vi "GT Axis Off.vi"(8 "error in (no error)":errorcluster caption="错误输入（无错误）", 10 "axis":i16, 11 "cardNum":i16) -> (0 "error out":errorcluster caption="错误输出", 3 "function return":i16)   [LabVIEW 2014, in "gts.lvlib"]
doc: "GT_API GT_AxisOff(short cardNum,short axis);"
uses:
  gts.lvlib
  gts.dll
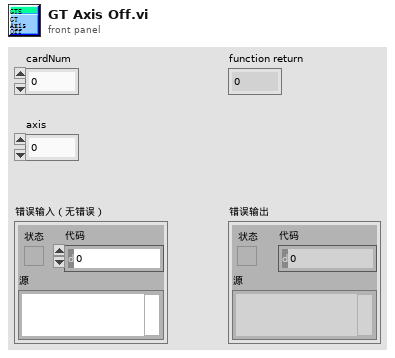
[diagram p1: front panel]
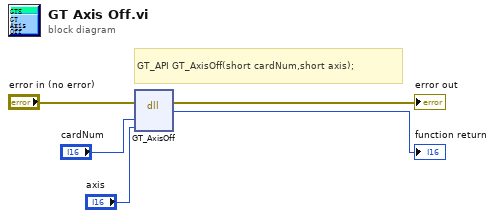
[diagram p0: block diagram]
diagram:
  # "GT_API GT_AxisOff(short cardNum,short axis);"
  n1 = dll-call lib="PTH2>abs F.多卡库-控制卡基本运动例程(labview)gts.*" fn="GT_AxisOff"(error in="error in (no error)", "cardNum"="cardNum", "axis"="axis") -> (error out=→"error out":errorcluster, →"function return":i16)  [unwired: 4 in, 1 out]
